vi "Module Init.vi"(8 "error in (no error)":errorcluster, 11 "HTTP Manager in":refnum<class "HTTP Manager.lvclass">) -> (0 "error out":errorcluster, 3 "HTTP Manager out":refnum<class "HTTP Manager.lvclass">)   [LabVIEW 2020, in "Volatus.lvlib" / "HTTP Manager.lvclass"]
uses:
  HTTP Manager.lvclass
  HTTP Manager.lvclass/HTTP Manager.ctl
  Module/Module.lvclass
  VolatusAPI/VolatusAPI.lvclass
  C:/dev/lv20CE/relink/lv-volatus/Volatus/Module/Module.lvclass
  C:/dev/lv20CE/relink/lv-volatus/Volatus/HTTP Manager/HTTP Manager.lvclass
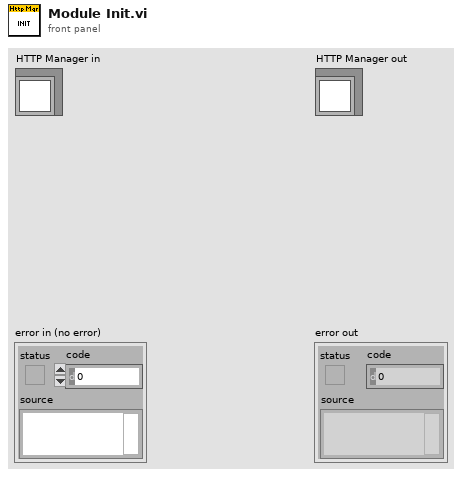
[diagram p1: front panel]
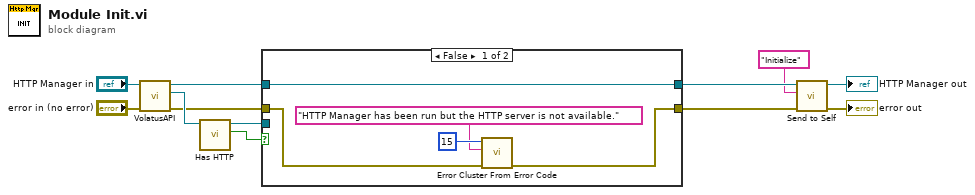
[diagram p0: block diagram]
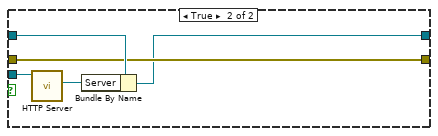
[diagram p2: hidden frame]
diagram:
  n1 = call "VolatusAPI.vi"("Module in"="HTTP Manager in") -> ("VolatusAPI"=w10:refnum<class "VolatusAPI.lvclass">, "Module out"=w6:refnum<class "HTTP Manager.lvclass">)  [unwired: 9 in]
  n2 = call "Has HTTP.vi"("VolatusAPI in"=w10) -> ("Has HTTP"=w9:bool, "VolatusAPI out"=w8:refnum<class "VolatusAPI.lvclass">)  [unwired: 9 in]
  n3 = case shown="False" w9 {
    tunnel: w8 -> [_ w21]
    tunnel: "error in (no error)" -> [w14 w18]
    tunnel: w6 -> [w16 w20]
    tunnel: [w12 w18] -> w5
    tunnel: [w16 w17] -> w3
    frame False {
      n4 = call <vilib>:"Error Cluster From Error Code.vi"("error in (no error)"=w14, "error message (\"\")"="HTTP Manager has been run but the HTTP server is not available.", "error code (0)"=15) -> ("error out"=w12:errorcluster)  [unwired: 6 in]
    }
    frame True {
      n5 = call "HTTP Server.vi"("VolatusAPI in"=w21) -> ("HTTP"=w19:refnum<class "Server.lvclass">)  [unwired: 9 in, 1 out]
      n6 = Bundle By Name(cluster=w20, "Server"=w19) -> (w17:refnum<class "HTTP Manager.lvclass">)
    }
  }
  n7 = call "Send to Self.vi"("error in (no error)"=w5, "Message ID"="Initialize", "Module in"=w3) -> ("error out"=→"error out":errorcluster, "Module out"=→"HTTP Manager out":refnum<class "HTTP Manager.lvclass">)  [unwired: 7 in]
